vi "ESA-C Correct Set Voltage.vi"(1 "Axis":i32, 2 "Target Voltage (V)":dbl) -> (0 "Command Voltage (V)":dbl)   [LabVIEW 2010]
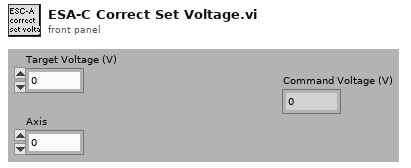
[diagram p1: front panel]
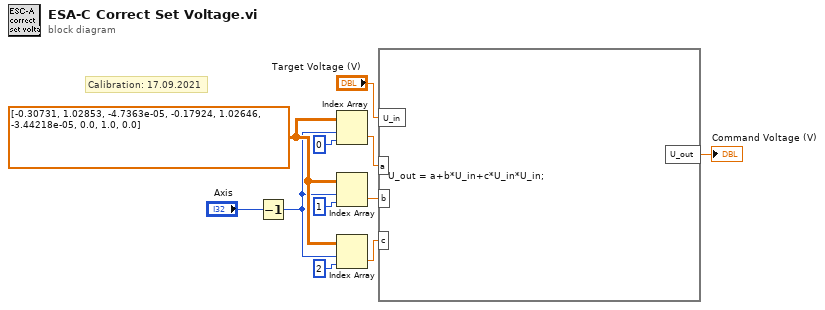
[diagram p0: block diagram]
diagram:
  w8 = dbl[][] [[-0.30731, 1.02853, -4.7363e-05], [-0.17924, 1.02646, -3.44218e-05], [0.0, 1.0, 0.0]]
  # "Calibration: 17.09.2021"
  n1 = Decrement(x="Axis") -> (x-1=w7:i32)
  n2 = Index Array(array=w8, index (row)=w7, index (col)=0 ("disabled index (col)")) -> (element=w3:dbl)
  n3 = Index Array(array=w8, index (row)=w7, index (col)=1 ("disabled index (col)")) -> (element=w2:dbl)
  n4 = Index Array(array=w8, index (row)=w7, index (col)=2 ("disabled index (col)")) -> (element=w1:dbl)
  n5 = formula code="U_out = a+b*U_in+c*U_in*U_in;"("U_in"="Target Voltage (V)", "a"=w3, "b"=w2, "c"=w1) -> ("U_out"=→"Command Voltage (V)":dbl)
